vi "RT_Incremental_Encoder_Main.vi"(8 "distance/count":dbl=9.38, 9 "Encoder Pins":T1(ring), 10 "Velocity Interval (uSec)":u32=1000) -> ()   [LabVIEW 2019]
uses:
  <vilib>/rvi/interface/nirviReadWriteControl/nirviReadWriteControl.xnode
  <vilib>/rvi/interface/nirviOpenFPGA/nirviOpenFPGA.xnode
  <vilib>/rvi/interface/nirviCloseFPGA/nirviCloseFPGA.xnode
  NiFpgaLv.dll
  <vilib>/Utility/error.llb/Error Cluster From Error Code.vi
  <vilib>/rvi/interface/Simulation/niFpgaSimulationCallBeginRW.vi
  <vilib>/rvi/errors/niLvFpgaAdjustHostInterfaceError.vi
  FPGA Bitfiles/gpass2_FPGATarget_FPGAIncremenalEn_kM8J46EtDIk.lvbitx
  FPGA_Incremental_Enc.vi
  <vilib>/FPGAPlugInAG/myRIO-1900/niLvFpga_Open_myRIO-1900.vi
  <vilib>/rvi/interface/common/dynamic/niFpgaDynamicAddResources.vi
  <vilib>/FPGAPlugInAG/Dynamic/niLvFpga_Close_Dynamic.vi
panel:
  out "Waveform Chart":dbl(graph)
  out "Acceleration [length/time^2]":dbl format="%.2f"
  out "Velocity [length/time]":dbl format="%.2f"
  out "Position [length]":dbl format="%.2f"
  out "Acceleration (Counts/Interval)":i32
  out "Velocity (Counts/Interval)":i32
  out "Position (Counts)":i64
  in  "Position Reset":bool
  in  "Loop Timer DAQ":u32=1
  in  "stop":bool
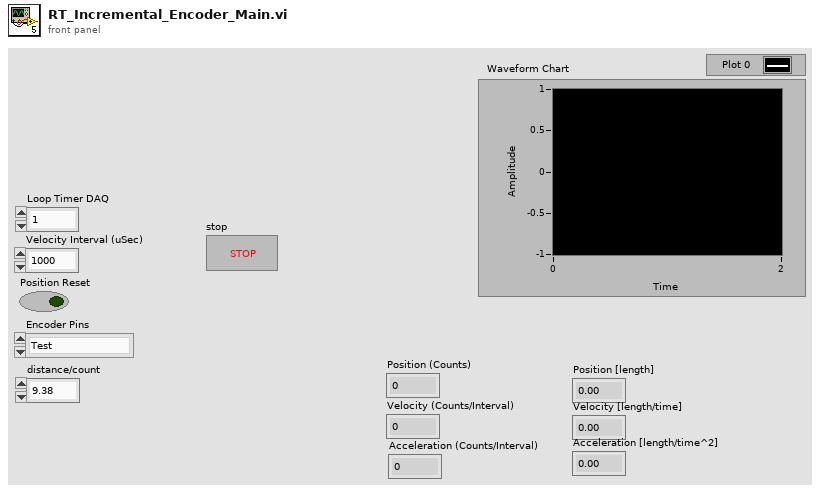
[diagram p1: front panel]
types:
  T1 = enum16{"Test", "Linear 1", "Linear 2", "Rotor 1", "Rotor 2"}
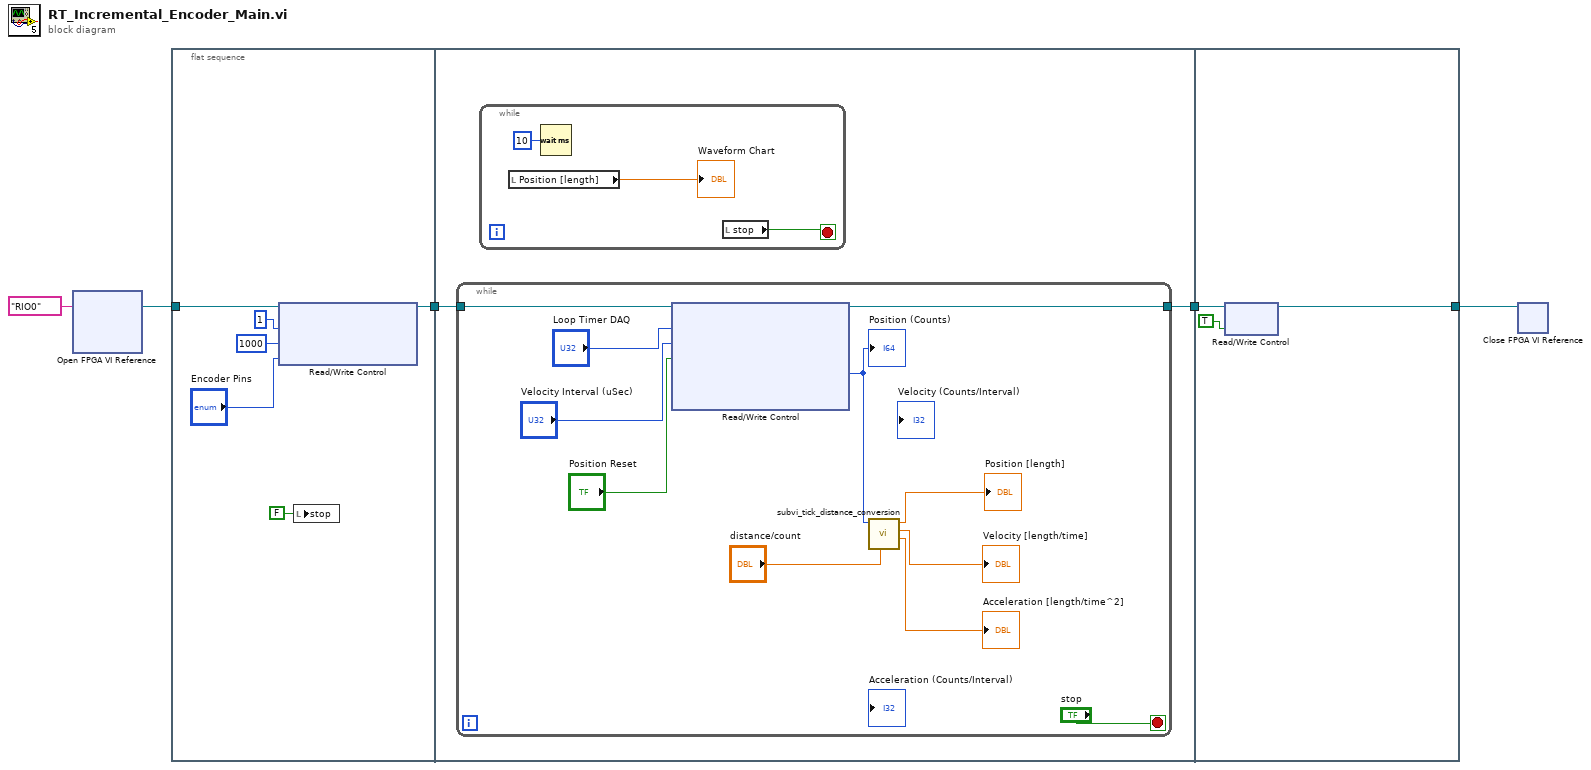
[diagram p0: block diagram]
diagram:
  n1 = xnode "Open FPGA VI Reference"("resource name"=tag "RIO0") -> ("FPGA VI Reference Out"=w4:refnum<k20>)  [unwired: 1 in, 1 out]
  n2 = flat-sequence {
    tunnel: w4 -> [w11]
    tunnel: [w8] -> w3
    tunnel: w3 -> [w13]
    tunnel: [w12] -> w2
    tunnel: w2 -> [w29]
    tunnel: [w28] -> w1
    frame #0 {
      n3 = xnode "Read/Write Control"("FPGA VI Reference In"=w11, "Loop Timer DAQ"=u32 1, "Velocity Interval (uSec)"=u32 1000, "Encoder Pins"="Encoder Pins") -> ("FPGA VI Reference Out"=w8:refnum<k20>)  [unwired: 1 in, 1 out]
      n4 = local write "stop"(FALSE ("stop")) -> ()
    }
    frame #1 {
      n5 = while {
        tunnel: w13 -> [w26]
        tunnel: [w22] -> w12
        stop <- "stop" stop-if-true
        n6 = xnode "Read/Write Control"("FPGA VI Reference In"=w26, "Loop Timer DAQ"="Loop Timer DAQ", "Velocity Interval (uSec)"="Velocity Interval (uSec)", "Position Reset"="Position Reset") -> ("FPGA VI Reference Out"=w22:refnum<k20>, "Position (Counts)"=w21:i64)  [unwired: 1 in, 3 out]
        "Position (Counts)" <- w21
        n7 = call "subvi_tick_distance_conversion.vi"("distance/count"="distance/count", "Position (Counts)"=w21) -> ("Acceleration [length/time^2]"=→"Acceleration [length/time^2]":dbl, "Velocity [length/time]"=→"Velocity [length/time]":dbl, "Position [length]"=→"Position [length]":dbl)  [unwired: 7 in]
      }
      n8 = while {
        stop <- w15 stop-if-true
        n9 = local read "Position [length]"() -> (→"Waveform Chart":dbl)
        n10 = Wait (ms)(milliseconds to wait=u32 10) -> ()  [unwired: 1 out]
        n11 = local read "stop"() -> (w15:bool)
      }
    }
    frame #2 {
      n12 = xnode "Read/Write Control"("FPGA VI Reference In"=w29, "stop"=TRUE) -> ("FPGA VI Reference Out"=w28:refnum<k20>)  [unwired: 1 in, 1 out]
    }
  }
  n13 = xnode "Close FPGA VI Reference"("FPGA VI Reference In"=w1) -> ()  [unwired: 1 in, 1 out]
